vi "Build Map.vi"(8 "error in (no error)":errorcluster, 11 "Map Model in":refnum<class "Map Model.lvclass">) -> (0 "error out":errorcluster, 3 "Map Model out":refnum<class "Map Model.lvclass">)   [LabVIEW 2020, in "Map Model.lvlib" / "Map Model.lvclass"]
uses:
  Map Model.lvclass
  Map Model.lvclass/Map Model.ctl
  <vilib>/picture/picture.llb/Draw 4-Bit Pixmap.vi
panel:
  # "NOTICE -- YOU MUST LEAVE THIS NOTICE IN PLACE.\n\nCopyright (c) 2017, LIANG LIU Shawn.Liu.cn@gmail.com\nAll rights reserved.\n\nRedistribution and use in source and binary forms, with or without modification, are permitted provided that the following conditions are met:\n-Redistributions of source code must retain the above copyright notice, this list of conditions and the following disclaimer.\n-Redistributions in binary form must reproduce the above copyright notice, this list of conditions and the following disclaimer in the documentation and/or other materials provided with the distribution.\n-Neither the name of the eLp nor the names of its contributors may be used to endorse or promote products derived from this software without specific prior written permission.\n\nTHIS SOFTWARE IS PROVIDED BY THE COPYRIGHT HOLDERS AND CONTRIBUTORS \"AS IS\" AND ANY EXPRESS OR IMPLIED WARRANTIES, INCLUDING, BUT NOT LIMITED TO, THE IMPLIED WARRANTIES OF MERCHANTABILITY AND FITNESS FOR A PARTICULAR PURPOSE ARE DISCLAIMED. IN NO EVENT SHALL THE COPYRIGHT HOLDER OR CONTRIBUTORS BE LIABLE FOR ANY DIRECT, INDIRECT, INCIDENTAL, SPECIAL, EXEMPLARY, OR CONSEQUENTIAL DAMAGES (INCLUDING, BUT NOT LIMITED TO, PROCUREMENT OF SUBSTITUTE GOODS OR SERVICES; LOSS OF USE, DATA, OR PROFITS; OR BUSINESS INTERRUPTION) HOWEVER CAUSED AND ON ANY THEORY OF LIABILITY, WHETHER IN CONTRACT, STRICT LIABILITY, OR TORT (INCLUDING NEGLIGENCE OR OTHERWISE) ARISING IN ANY WAY OUT OF THE USE OF THIS SOFTWARE, EVEN IF ADVISED OF THE POSSIBILITY OF SUCH DAMAGE."
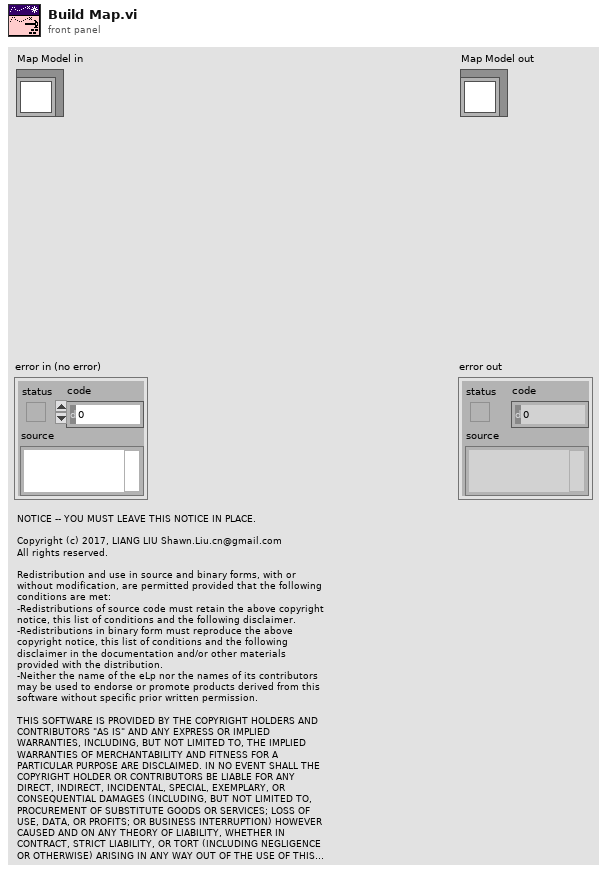
[diagram p1: front panel]
types:
  T1 = cluster{"Occupied Color":cluster{"Value":u8, "Color":u32}, "Free Color":cluster{"Value":u8, "Color":u32}, "Unknown Color":cluster{"Value":u8, "Color":u32}}
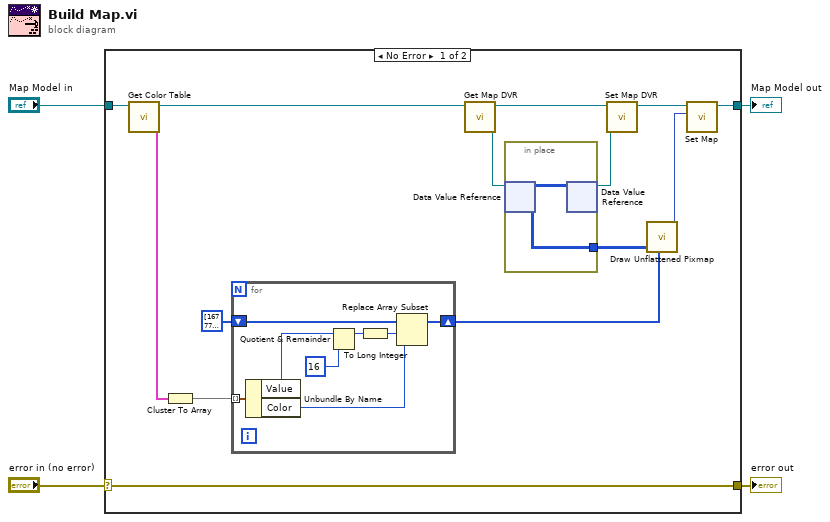
[diagram p0: block diagram]
diagram:
  n1 = case shown="No Error" "error in (no error)" {
    selector: "error in (no error)" -> [w7 w29]
    tunnel: "Map Model in" -> [w11 w28]
    tunnel: [w6 w28] -> w2
    tunnel: [w7 w29] -> w1
    frame No Error {
      n2 = call "Get Color Table.vi"("Map Model in"=w11) -> ("Color Table"=w13:T1, "Map Model out"=w10:refnum<class "Map Model.lvclass">)  [unwired: 9 in]
      n3 = Cluster To Array(cluster=w13) -> (array=w12:cluster{"Value":u8, "Color":u32}[])
      n4 = for {
        shift-right: [w25] -> w9
        shift-left: u32[] [16777215, 16776960, 128, 16711680, 16711935, 8388736, 255, 65535, 65280, 32768, 8388608, 8421376, 12632256, 8421504, 32896, 0] ("color table") -> [w26]
        tunnel: w12 -> [w24] mode=indexing
        n5 = Unbundle By Name(w24) -> ("Value"=w23:u8, "Color"=w21:u32)
        n6 = Quotient & Remainder(x=w23, y=u8 16) -> (x-y*floor(x/y)=w22:u8)  [unwired: 1 out]
        n7 = To Long Integer(number=w22) -> (32bit integer=w20:i32)
        n8 = Replace Array Subset(array=w26, new element=w21, index=w20) -> (w25:u32[])
      }
      n9 = call "Get Map DVR.vi"("Map Model in"=w10) -> ("Map DVR"=w16:refnum<data-value>, "Map Model out"=w18:refnum<class "Map Model.lvclass">)  [unwired: 9 in]
      n10 = in-place {
        in-place-border: [w27] -> w15
        n11 = in-place-dvr #1(w16) -> (w27:u8[][])  [unwired: 1 out]
        n12 = in-place-dvr #1(w27) -> (w17:refnum<data-value>)  [unwired: 1 out]
      }
      n13 = call "Set Map DVR.vi"("Map DVR"=w17, "Map Model in"=w18) -> ("Map Model out"=w8:refnum<class "Map Model.lvclass">)  [unwired: 9 in]
      n14 = call-poly <vilib>:"Draw Unflattened Pixmap.vi"("data"=w15, "color table"=w9) -> ("new picture"=w5:picture)  [unwired: 7 in]
      n15 = call "Set Map.vi"("Map"=w5, "Map Model in"=w8) -> ("Map Model out"=w6:refnum<class "Map Model.lvclass">)  [unwired: 9 in]
    }
    frame Error {
    }
  }
  "error out" <- w1
  "Map Model out" <- w2
